vi "Set File Renum.vi"(2 "error in":errorcluster, 3 "file name":string) -> (0 "error out":errorcluster, 1 "file refnum":refnum<file>)   [LabVIEW 2016]
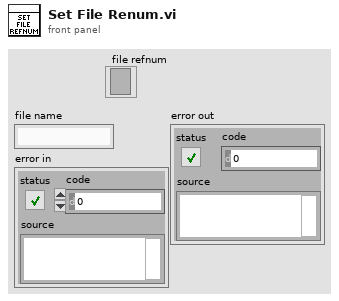
[diagram p1: front panel]
types:
  T1 = enum16{"open", "replace", "create", "open or create", "replace or create", "replace or create with confirmation"}
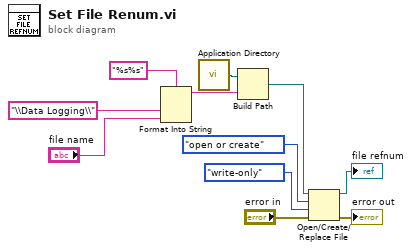
[diagram p0: block diagram]
diagram:
  n1 = Format Into String(format string="%s%s", "\\Data Logging\\", "file name") -> (resulting string=w7:string)  [unwired: 2 in, 1 out]
  n2 = call <vilib>:"Application Directory.vi"() -> ("Application Directory"=w11:path)
  n3 = Build Path(base path=w11, name or relative path=w7) -> (appended path=w6:path)
  n4 = Open/Create/Replace File(file path (use dialog)=w6, error in="error in", operation (0:open)=T1."open or create", access (0:read/write)=enum16{"read/write", "read-only", "write-only"}."write-only") -> (refnum out=→"file refnum":refnum<file>, error out=→"error out":errorcluster)  [unwired: 2 in, 1 out]
